vi "Retrieve Bus A Raw Log.vi"(5 "Component ID":u8, 7 "FPGA Interface":refnum<class "FPGA Interface.lvclass">, 8 "error in (no error)":errorcluster, 11 "Bus Monitor in":refnum<class "Bus Monitor.lvclass">) -> (0 "error out":errorcluster, 2 "Bus A Raw Log":u16[](array[numeric]) format="%.0x", 3 "Bus Monitor out":refnum<class "Bus Monitor.lvclass">)   [LabVIEW 2016, in "BCI-1553 API.lvlib" / "Bus Monitor.lvclass"]
doc: "Retrieves and loosely organizes the contents of the Bus A monitor buffer."
uses:
  Bus Monitor.lvclass
  TypeDefs/Bus Monitor Read Config.ctl
  Dependencies/FPGA Interface/FPGA Interface.lvclass
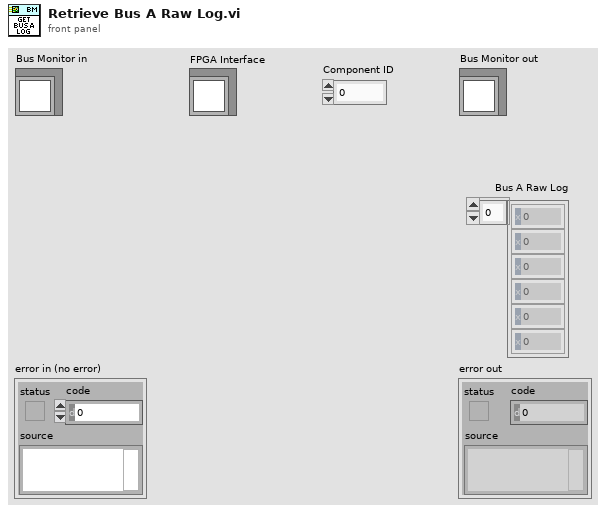
[diagram p1: front panel]
types:
  T1 = typedef "BCI-1553 API.lvlib/Bus Monitor.lvclass/Bus Monitor Read Config.ctl" = cluster{"cmdRecordStart":u16, "cmdRecordLength":u16, "dataRecordStart":u16, "dataRecordEnd":u16}
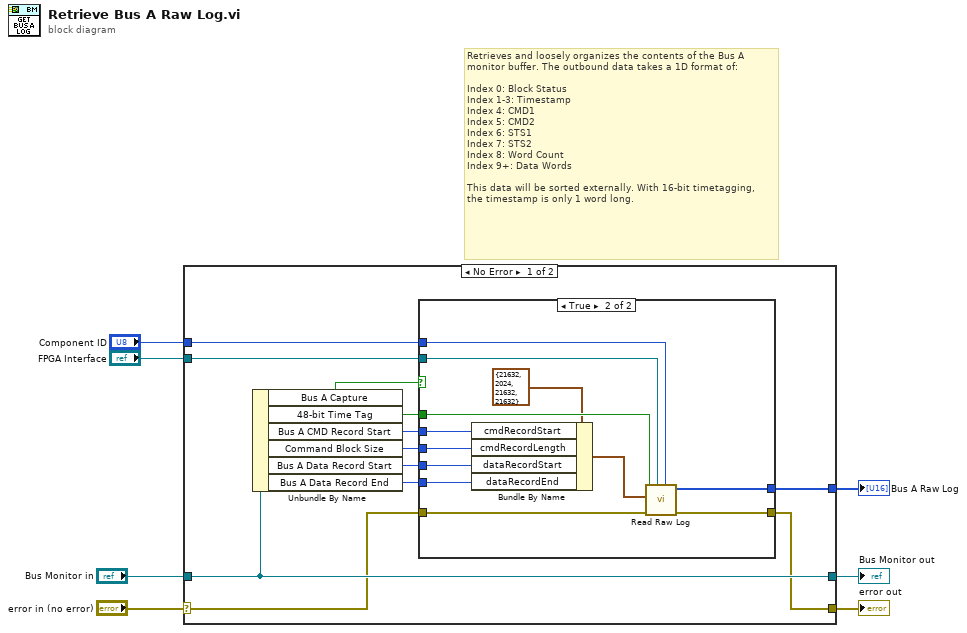
[diagram p0: block diagram]
diagram:
  # "Retrieves and loosely organizes the contents of the Bus A\nmonitor buffer. The outbound data takes a 1D format of:\n\nIndex 0: Block Status\nIndex 1-3: Timestamp\nIndex 4: CMD1\nIndex 5: CMD2\nIndex 6: STS1\nIndex 7: STS2\nIndex 8: Word Count\nIndex 9+: Data Words\n\nThis data will be sorted externally. With 16-bit timetagging,\nthe timestamp is only 1 word long."
  n1 = case shown="No Error" "error in (no error)" {
    selector: "error in (no error)" -> [w10 w33]
    tunnel: [w15 w33] -> w6
    tunnel: [w16 w32] -> w4
    tunnel: "Bus Monitor in" -> [w16 w32]
    tunnel: [w19 _] -> w3
    tunnel: "FPGA Interface" -> [w18 _]
    tunnel: "Component ID" -> [w17 _]
    frame No Error {
      n2 = Unbundle By Name(w16) -> ("Bus A Capture"=w11:bool, "48-bit Time Tag"=w12:bool, "Bus A CMD Record Start"=w13:u16, "Command Block Size"=w14:u16, "Bus A Data Record Start"=w9:u16, "Bus A Data Record End"=w8:u16)
      n3 = case shown="True" w11 {
        tunnel: [_ w27] -> w19
        tunnel: w18 -> [_ w29]
        tunnel: w17 -> [_ w28]
        tunnel: [_ w26] -> w15
        tunnel: w14 -> [_ w22]
        tunnel: w13 -> [_ w23]
        tunnel: w12 -> [_ w30]
        tunnel: w10 -> [_ w31]
        tunnel: w9 -> [_ w21]
        tunnel: w8 -> [_ w20]
        frame False {
        }
        frame True {
          n4 = Bundle By Name(cluster=T1 {"cmdRecordStart"=21632, "cmdRecordLength"=2024, "dataRecordStart"=21632, "dataRecordEnd"=21632} ("bmReadConfig"), "cmdRecordStart"=w23, "cmdRecordLength"=w22, "dataRecordStart"=w21, "dataRecordEnd"=w20) -> (w24:T1)
          n5 = call "Read Raw Log.vi"("Component ID"=w28, "FPGA Interface"=w29, "error in (no error)"=w31, "bmReadConfig"=w24, "48-bit Timetag?"=w30) -> ("error out"=w26:errorcluster, "Raw Log"=w27:u16[])  [unwired: 5 in]
        }
      }
    }
    frame Error {
    }
  }
  "error out" <- w6
  "Bus Monitor out" <- w4
  "Bus A Raw Log" <- w3
